vi "Read Movie File Header (SubVI).vi"(11 "File Name":path) -> (2 "Array":u64[](array[numeric]), 3 "Movie File REF":refnum<file>)   [LabVIEW 2015]
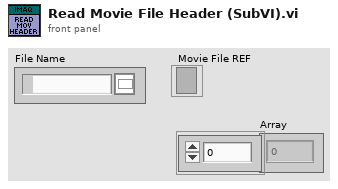
[diagram p1: front panel]
types:
  T1 = enum16{"big-endian, network order", "native, host order", "little-endian"}
  T2 = enum16{"open", "replace", "create", "open or create", "replace or create", "replace or create with confirmation"}
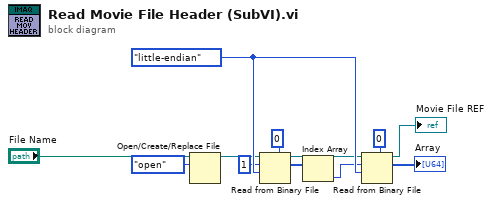
[diagram p0: block diagram]
diagram:
  w10 = T1."little-endian" ("byte order (0:big-endian, network order)")
  n1 = Open/Create/Replace File(file path (use dialog)="File Name", operation (0:open)=T2."open") -> (refnum out=w9:refnum<file>)  [unwired: 4 in, 2 out]
  n2 = Read from Binary File(5:0 ("count (1)"), 9:w10, 10:1 ("count (1)"), 11:w9) -> (2:w4:i32[], 3:w5:refnum<file>)  [unwired: 2 in, 2 out]
  n3 = Index Array(array=w4) -> (element=w3:i32)  [unwired: 1 in]
  n4 = Read from Binary File(5:u64 0 ("count (1)"), 9:w10, 10:w3, 11:w5) -> (2:→"Array":u64[], 3:→"Movie File REF":refnum<file>)  [unwired: 2 in, 2 out]
